vi "generate table.vi"(5 "to tbwi":refnum<vi>, 6 "Direction":enum32{"From TBWI", "To TBWI"}(radio), 7 "from tbwi":refnum<vi>, 8 "error in":errorcluster, 9 "tags":refnum<vi>, 10 "engine configuration in":refnum<class "engine configuration.lvclass">, 11 "Tag Bus Web Interface configuration in":refnum<class "Tag Bus Web Interface configuration.lvclass">) -> (0 "error out":errorcluster, 3 "TBWI Cfg out":refnum<class "Tag Bus Web Interface configuration.lvclass">)   [LabVIEW 2013, in "Tag Bus Web Interface editor node.lvclass"]
uses:
  Tag Bus Web Interface editor node.lvclass
  configuration/Tag Bus Web Interface configuration.lvclass
  <vilib>/NI/Module Execution Interface/Engine Configuration/engine configuration.lvclass
  <vilib>/NI/Configuration Framework/serializable configuration/NISE_CEF_serializable configuration.lvclass/NISE_CEF_serializable configuration.ctl
  configuration/Tag Bus Web Interface configuration.lvclass/Tag Bus Web Interface configuration.ctl
  <vilib>/NI/Tag Bus/tag/tag descriptor.lvclass/tag descriptor.ctl
  <vilib>/NI/Tag Bus Module Framework/channel/channel classification.ctl
  <vilib>/NI/Tag Bus Module Framework/channel/TBM channel.lvclass/TBM channel.ctl
  <vilib>/NI/Module Execution Interface/Engine Configuration/engine configuration.lvclass/engine configuration.ctl
  <vilib>/NI/Tag Bus/tag/read tag name.vi
  <vilib>/NI/Tag Bus Module Framework/channel/Read channel classification.vi
  <vilib>/NI/Tag Bus/tag/read data type.vi
  <vilib>/NI/Configuration Framework/serializable configuration/Read UID.vi
  configuration/Read channels.vi
  <vilib>/Utility/LVClass/Get LV Class Name.vi
  <vilib>/NI/Configuration Framework/error generator/NISE_error generator.vi
  <vilib>/NI/Tag Bus Module Framework/channel/TBM channel.lvclass
  <vilib>/NI/Tag Bus/tag/tag descriptor.lvclass
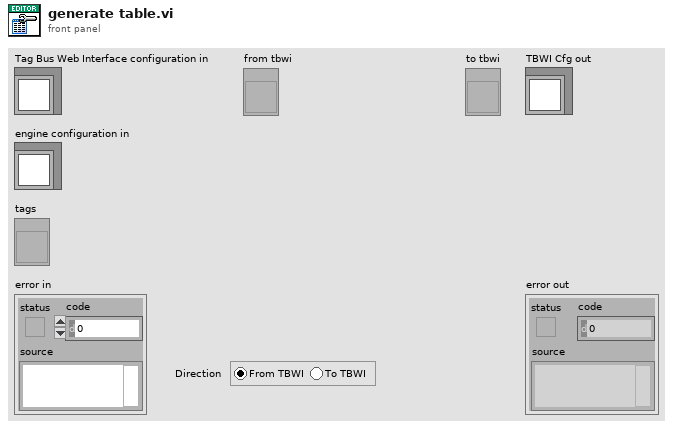
[diagram p1: front panel]
types:
  T1 = typedef "tag bus.lvlib/tag descriptor.lvclass/Data Type.ctl" = enum16{"Double", "Single", "I64", "I32", "I16", "I8", "U64", "U32", "U16", "U8", "Boolean", "String", "Array of Double", "Array of Single", "Array of I64", "Array of I32", "Array of I16", "Array of I8", "Array of U64", "Array of U32", "Array of U16", "Array of U8", "Array of Boolean", "Array of String"}
  T2 = typedef "TBM channel.lvclass/channel classification.ctl" = enum16{"input data", "output data", "processing parameter", "processing result"}
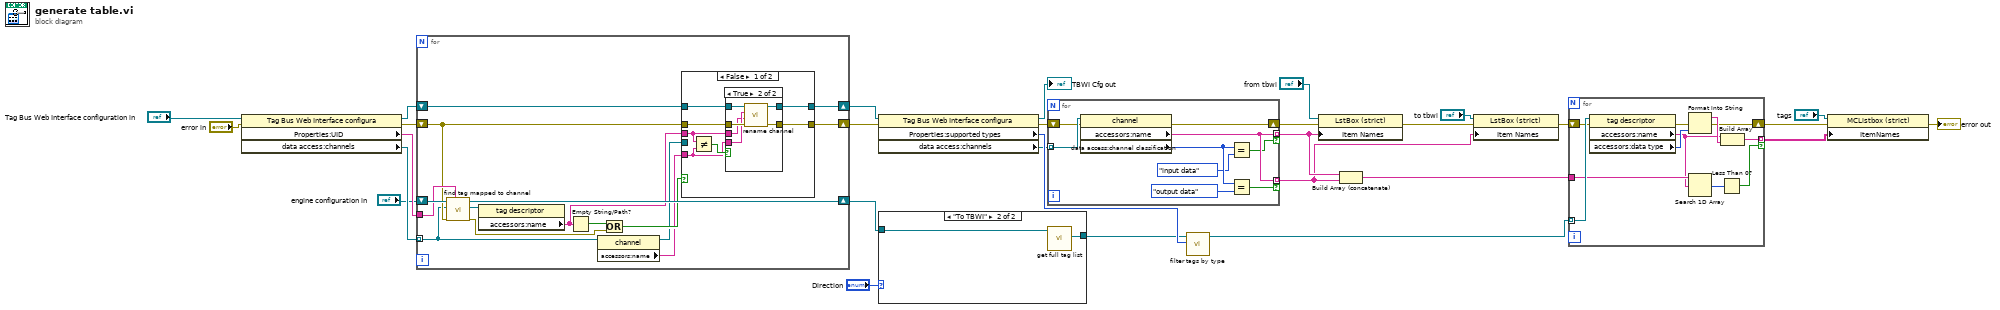
[diagram p0: block diagram]
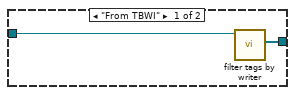
[diagram p2: hidden frame]
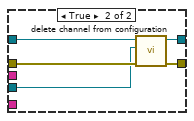
[diagram p4: hidden frame]
diagram:
  n1 = property class="Tag Bus Web Interface configura"(reference="Tag Bus Web Interface configuration in", error in="error in") -> (reference out=w27:refnum<class "Tag Bus Web Interface configuration.lvclass">, error out=w28:errorcluster, "Properties:UID"=w23:string, "data access:channels"=w29:refnum<class "TBM channel.lvclass">[])
  n2 = for {
    tunnel: w29 -> [w34] mode=indexing
    shift-right: [w42] -> w15
    shift-left: "engine configuration in" -> [w44]
    shift-right: [w39] -> w26
    shift-left: w27 -> [w37]
    tunnel: w23 -> [w43]
    shift-right: [w38] -> w25
    shift-left: w28 -> [w35]
    n3 = call <vilib>:"find tag mapped to channel.vi"("owner"=w43, "error in"=w35, "channel"=w34, "engine configuration in"=w44) -> ("error out"=w33:errorcluster, "tag"=w41:refnum<class "tag descriptor.lvclass">, "engine configuration out"=w42:refnum<class "engine configuration.lvclass">)  [unwired: 5 in]
    n4 = property class="tag descriptor"(reference=w41) -> ("accessors:name"=w31:string)  [unwired: 1 in, 2 out]
    n5 = Empty String/Path?(string/path=w31) -> (empty?=w40:bool)
    n6 = property class="channel"(reference=w34) -> (reference out=w30:refnum<class "TBM channel.lvclass">, "accessors:name"=w32:string)  [unwired: 1 in, 1 out]
    n7 = Or(x=w40, y=w33) -> (x .or. y?=w36:bool)
    n8 = case shown="False" w36 {
      tunnel: [w48 w64] -> w39
      tunnel: [w51 w63] -> w38
      tunnel: w35 -> [w50 w62]
      tunnel: w37 -> [w49 w61]
      tunnel: w32 -> [w46 _]
      tunnel: w31 -> [w45 _]
      tunnel: w30 -> [_ w60]
      frame False {
        n9 = Not Equal?(x=w45, y=w46) -> (x != y?=w47:bool)
        n10 = case shown="True" w47 {
          tunnel: [w53 w58] -> w51
          tunnel: w50 -> [w53 w59]
          tunnel: w49 -> [w52 w57]
          tunnel: [w52 w56] -> w48
          tunnel: w46 -> [_ w55]
          tunnel: w45 -> [_ w54]
          frame False {
          }
          frame True {
            n11 = call "rename channel.vi"("error in"=w59, "new name"=w54, "old name"=w55, "Tag Bus Web Interface configuration in"=w57) -> ("error out"=w58:errorcluster, "Tag Bus Web Interface configuration out"=w56:refnum<class "Tag Bus Web Interface configuration.lvclass">)  [unwired: 6 in]
          }
        }
      }
      frame True {
        n12 = call "delete channel from configuration.vi"("error in"=w62, "TBM channel in"=w60, "Tag Bus Web Interface configuration in"=w61) -> ("error out"=w63:errorcluster, "Tag Bus Web Interface configuration out"=w64:refnum<class "Tag Bus Web Interface configuration.lvclass">)  [unwired: 7 in]
      }
    }
  }
  n13 = property class="Tag Bus Web Interface configura"(reference=w26, error in=w25) -> (reference out=→"TBWI Cfg out":refnum<class "Tag Bus Web Interface configuration.lvclass">, error out=w21:errorcluster, "Properties:supported types"=w24:T1[], "data access:channels"=w22:refnum<class "TBM channel.lvclass">[])
  n14 = case shown="\"To TBWI\"" "Direction" {
    tunnel: w15 -> [w66 w68]
    tunnel: [w65 w67] -> w14
    frame "From TBWI" {
      n15 = call <vilib>:"filter tags by writer.vi"("engine configuration in"=w66) -> ("tag list"=w65:refnum<class "tag descriptor.lvclass">[])  [unwired: 9 in, 1 out]
    }
    frame "To TBWI" {
      n16 = call <vilib>:"get full tag list.vi"("engine configuration in"=w68) -> ("tag list"=w67:refnum<class "tag descriptor.lvclass">[])  [unwired: 9 in, 1 out]
    }
  }
  n17 = for {
    tunnel: w22 -> [w77] mode=indexing
    shift-right: [w76] -> w13
    shift-left: w21 -> [w75]
    tunnel: [w74] -> w9 mode=indexing if=w72
    tunnel: [w74] -> w10 mode=indexing if=w71
    n18 = property class="channel"(reference=w77, error in=w75) -> (error out=w76:errorcluster, "accessors:name"=w74:string, "data access:channel classification"=w73:T2)  [unwired: 1 out]
    n19 = Equal?(x=w73, y=channel_classification."input data") -> (x = y?=w71:bool)
    n20 = Equal?(x=w73, y=channel_classification."output data") -> (x = y?=w72:bool)
  }
  n21 = call <vilib>:"filter tags by type.vi"("allowable types"=w24, "tags in"=w14) -> ("filtered tags"=w20:refnum<class "tag descriptor.lvclass">[])  [unwired: 9 in]
  n22 = property class="LstBox (strict)"(reference="from tbwi", error in=w13, "Item Names"=w10) -> (error out=w12:errorcluster)  [unwired: 1 out]
  n23 = Build Array (concatenate)(w10, w9) -> (w8:string[])
  n24 = property class="LstBox (strict)"(reference="to tbwi", error in=w12, "Item Names"=w9) -> (error out=w19:errorcluster)  [unwired: 1 out]
  n25 = for {
    tunnel: w20 -> [w86] mode=indexing
    shift-right: [w83] -> w18
    shift-left: w19 -> [w85]
    tunnel: [w82] -> w17 mode=indexing if=w78
    tunnel: w8 -> [w81]
    n26 = property class="tag descriptor"(reference=w86, error in=w85) -> (error out=w84:errorcluster, "accessors:name"=w79:string, "accessors:data type"=w87:T1)  [unwired: 1 out]
    n27 = Format Into String(error in=w84, w87) -> (resulting string=w88:string, error out=w83:errorcluster)  [unwired: 2 in]
    n28 = Search 1D Array(1D array=w81, element=w79) -> (index of element=w80:i32)  [unwired: 1 in]
    n29 = Less Than 0?(x=w80) -> (x < 0?=w78:bool)
    n30 = Build Array(w79, w88) -> (w82:string[])
  }
  n31 = property class="MCListbox (strict)"(reference="tags", error in=w18, "ItemNames"=w17) -> (error out=→"error out":errorcluster)  [unwired: 1 out]
